vi "exec.vi"(8 "error in (no error)":errorcluster, 10 "context":refnum<class "IContextThisComponent.lvclass">, 11 "SetSpectTempSetpoint in":refnum<class "setSpectTempSetpoint.lvclass">) -> (0 "error out":errorcluster, 2 "context 2":refnum<class "IContextThisComponent.lvclass">, 3 "SetSpectTempSetpoint out":refnum<class "setSpectTempSetpoint.lvclass">)   [LabVIEW 2016, in "Commands.lvlib" / "setSpectTempSetpoint.lvclass"]
uses:
  setSpectTempSetpoint.lvclass
  IContextThisComponent/IContextThisComponent.lvclass
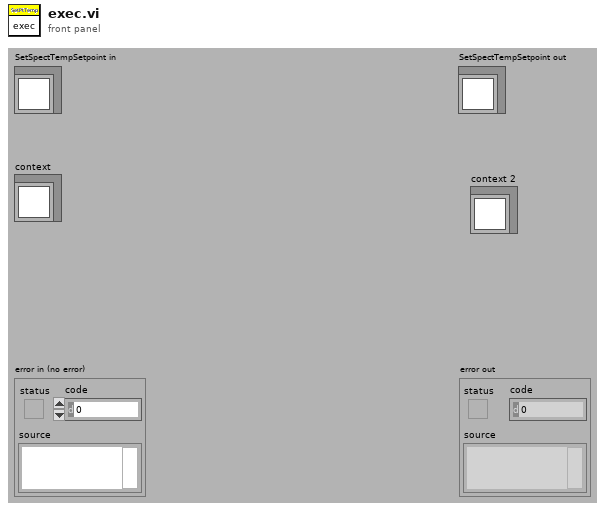
[diagram p1: front panel]
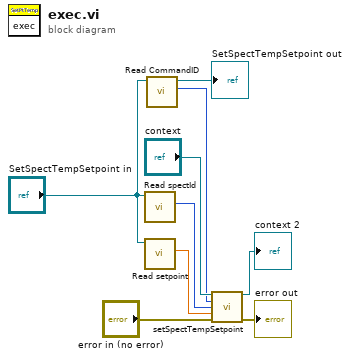
[diagram p0: block diagram]
diagram:
  n1 = call-dynamic "Read spectId.vi"("SetSpectTempSetpoint in"="SetSpectTempSetpoint in") -> ("spectId"=w1:u16)  [unwired: 8 in, 2 out]
  n2 = call-dynamic "Read setpoint.vi"("SetSpectTempSetpoint in"="SetSpectTempSetpoint in") -> ("setpoint"=w2:sgl)  [unwired: 8 in, 2 out]
  n3 = call-dynamic "Read CommandID.vi"("Command in"="SetSpectTempSetpoint in") -> ("CommandID"=w4:i32, "Command out"=→"SetSpectTempSetpoint out":refnum<class "setSpectTempSetpoint.lvclass">)  [unwired: 8 in, 1 out]
  n4 = call-dynamic "setSpectTempSetpoint.vi"("IContextThisComponent in"="context", "CommandID"=w4, "spectId"=w1, "setpoint"=w2, "error in (no error)"="error in (no error)") -> ("IContextThisComponent out"=→"context 2":refnum<class "IContextThisComponent.lvclass">, "error out"=→"error out":errorcluster)  [unwired: 9 in]
